vi "SimuladorTemp.vi"(1 "Lim Max T":dbl, 2 "Lim Min T":dbl) -> (0 "Numeric":dbl)   [LabVIEW 2020]
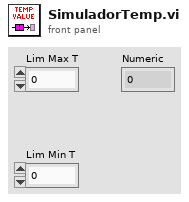
[diagram p1: front panel]
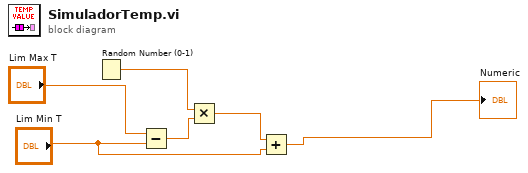
[diagram p0: block diagram]
diagram:
  n1 = Random Number (0-1)() -> (number: 0 to 1=w2:dbl)
  n2 = Subtract(x="Lim Max T", y="Lim Min T") -> (x-y=w3:dbl)
  n3 = Multiply(x=w2, y=w3) -> (x*y=w4:dbl)
  n4 = Add(x=w4, y="Lim Min T") -> (x+y=→"Numeric":dbl)
